vi "Encode Return Codes.vi"(10 "Subscription Success":T1[](array[typedef])) -> (2 "Return Codes":u8[](array[numeric]) format="%08b")   [LabVIEW 2013, in "SUBACK.lvclass"]
uses:
  SUBACK.lvclass
  Subscription Success Code.ctl
  ControlPacket/QualityOfService -- enum.ctl
  ControlPacket/ControlPacket.lvclass
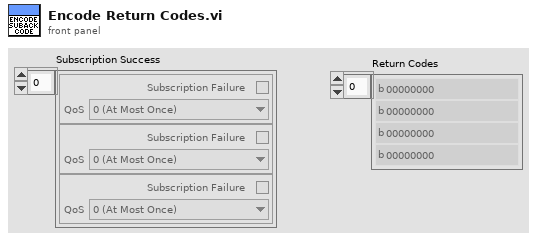
[diagram p1: front panel]
types:
  T1 = typedef "SUBACK.lvclass/Subscription Success Code.ctl" = cluster{"Subscription Failure":bool, "QoS":T2}
  T2 = typedef "ControlPacket.lvclass/QualityOfService -- enum.ctl" = enum16{"0 (At Most Once)", "1 (At Least Once)", "2 (Exactly Once)"}
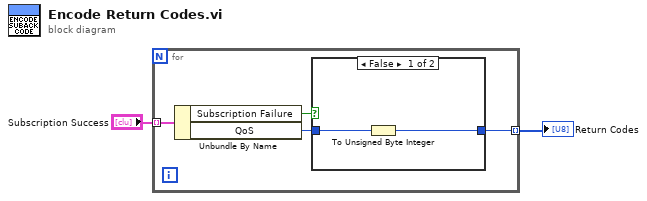
[diagram p0: block diagram]
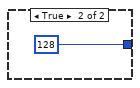
[diagram p2: hidden frame]
diagram:
  n1 = for {
    tunnel: "Subscription Success" -> [w6] mode=indexing
    tunnel: [w4] -> w1 mode=indexing
    n2 = Unbundle By Name(w6) -> ("Subscription Failure"=w3:bool, "QoS"=w5:T2)
    n3 = case shown="False" w3 {
      tunnel: w5 -> [w8 _]
      tunnel: [w7 u8 128 ("y")] -> w4
      frame False {
        n4 = To Unsigned Byte Integer(number=w8) -> (unsigned 8bit integer=w7:u8)
      }
      frame True {
      }
    }
  }
  "Return Codes" <- w1
